vi "Robot Global Data.vi"() -> ()   [LabVIEW 2014]
doc: "This global VI can contain as many global variables as you need. Place a control on the panel, give it a good name. To read or write to it from a VI, drag the icon to the diagram of that VI. You can also drag from the project. Click on the node to change which global you access. You shouldn't have multiple locations writing to a global or it will cause a race-condition."
uses:
  <vilib>/Rock Robotics/WPI/Camera/WPI_CameraImageSize.ctl
  <vilib>/Rock Robotics/WPI/DriverStation/WPI_DriverStationRobotMode2.ctl
panel:
  out "No Lift":bool
  out "Stabilizer Open":bool
  out "Stabilizer Close":bool
  out "RC Open":bool
  out "RC Close":bool
  out "Fast Lift":bool
  out "Cylinder Close":bool
  out "Cylinder Open":bool
  out "Lift Stop":bool
  out "Manual LIft":bool
  out "Slow Mode":bool
  out "Photoeye 5":bool
  out "Level Drive":bool
  out "Level Down":bool
  out "Level Up":bool
  out "Any Photoeye":bool
  out "Lift Down":bool
  out "Lift Up":bool
  out "Brake Time":u32
  out "Lift Drive":bool
  out "Photoeye 4":bool
  out "Photoeye 3":bool
  out "Photoeye 2":bool
  out "Photoeye 1":bool
  in  "Robot Mode":T1
  in  "image size":T2=enum."320x240"
  in  "Enable Vision":bool=TRUE
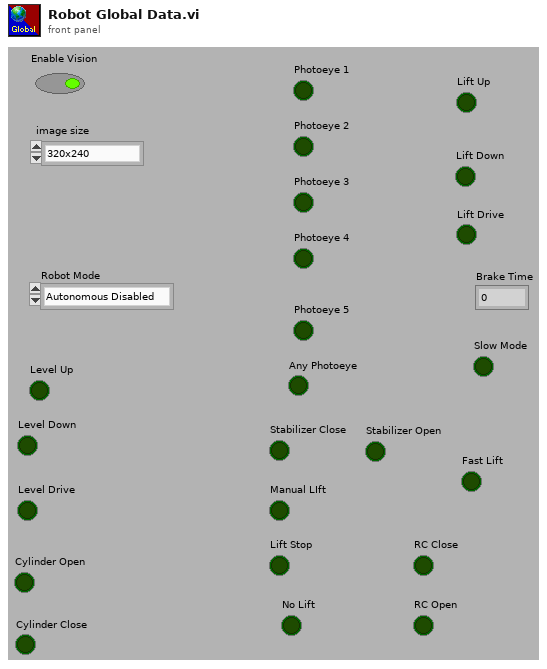
[diagram p1: front panel]
types:
  T1 = typedef "WPI_DriverStationRobotMode2.ctl" = enum16{"Autonomous Disabled", "Autonomous Enabled", "Teleop Disabled", "Teleop Enabled", "Disconnected", "Finish", "Test Disabled", "Test Enabled", "Emergency Stopped"}
  T2 = typedef "WPI_CameraImageSize.ctl" = enum16{"640x480", "320x240", "160x120", "Custom"}
diagram:
